vi "PID_controllerT_05.vi"() -> ()   [LabVIEW 2011]
uses:
  <vilib>/Platform/TimedLoop/XDataNode/nitl_modes.ctl
  <vilib>/Platform/TimedLoop/XDataNode/timing_clust.ctl
  <vilib>/Platform/TimedLoop/XDataNode/wakeup.ctl
  <vilib>/Platform/TimedLoop/XDataNode/XDataNode.xnode
  <vilib>/Platform/TimedLoop/XDataNode/XDNodeRunTimeDep.lvlib
panel:
  out "error(t-t0)":cluster{dbl, "Value":dbl}[](array[cluster])
  out "error":dbl
  out "tStart(s)":dbl
  out "x-y":dbl
  out "S00":dbl
  out "S10":dbl
  out "S20":dbl
  out "S11":dbl
  out "S01":dbl
  out "weight":dbl[](array[numeric])
  in  "# of points to watch":i32
  in  "tSmooth(s)":dbl=-1.0
  out "t0":dbl
  out "error(t)":cluster{dbl, "Value":dbl}[](array[cluster])
  out "error out":errorcluster
  out "first":bool=TRUE
  out "P (torr)":string
  out "XY Graph":cluster{dbl, "Value":dbl}[](graph)
  out "current value":dbl
  in  "stop":bool
  in  "Period (s)":dbl
  out "dValue":dbl
  out "derivative":dbl
  out "integral":dbl
  out "Current angle (deg)":dbl
  in  "Kd":dbl
  in  "Ki":dbl
  in  "Kp":dbl
  out "Current P (torr)":dbl
  in  "Set Point (torr)":dbl
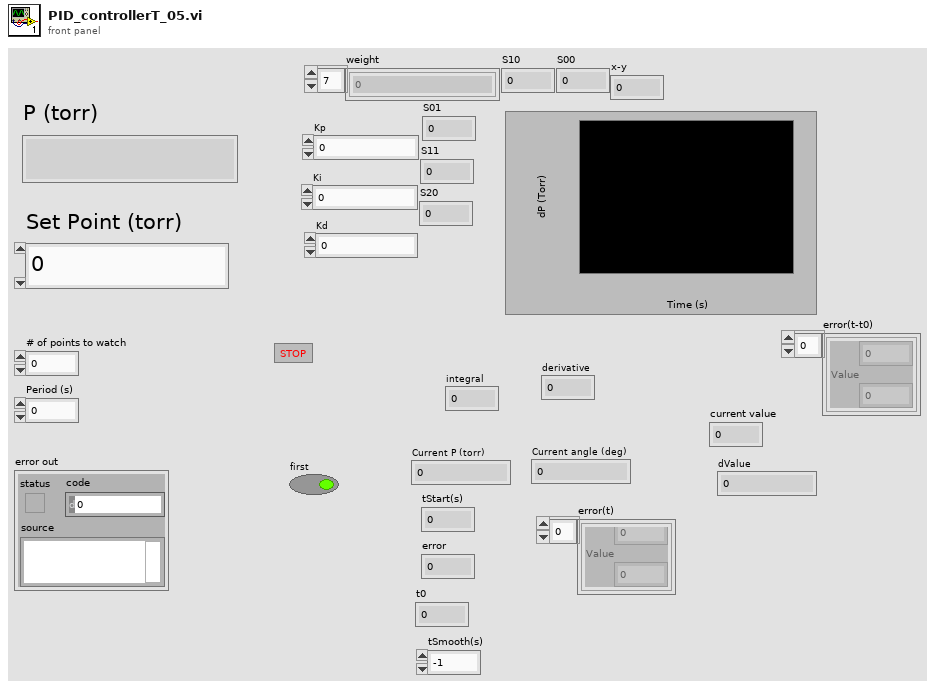
[diagram p1: front panel]
types:
  T1 = typedef "XDNodeRunTimeDep.lvlib/nitl_modes.ctl" = enum32{"No Change", "Process missed periods, maintain original phase", "Discard missed periods, maintain original phase", "Process missed periods, ignore original phase", "Discard missed periods, ignore original phase"}
  T2 = typedef "XDNodeRunTimeDep.lvlib/timing_clust.ctl" = cluster{"Expected End [f-1]":u64, "Actual End [f-1]":u64, "Finished Late? [f-1]":bool, "Expected End [i-1]":u64, "Actual End [i-1]":u64, "Finished Late? [i-1]":bool, "Expected Start [i]":u64, "Actual Start [i]":u64, "Expected Start [f]":u64, "Actual Start [f]":u64, "Source Name":string, "Structure Name":string, "Period":i64, "Deadline":i64, "Offset":i64, "Start":i64, "Priority":i32, "Timeout":i32, "Mode":T1, "Wakeup Reason":T3, "Error":errorcluster, "Source Type":string, "Secondary Source Type":string, "Global End Time":u64, "Global Start Time":u64, "Frame Duration":u64, "Iteration Duration":u64, "Assigned CPU":i32, "I/O Scan Engine Mode":u32}
  T3 = typedef "XDNodeRunTimeDep.lvlib/wakeup.ctl" = enum32{"Normal", "Aborted", "Asynchronous wakeup", "Timing source error", "Timed loop error", "Timeout"}
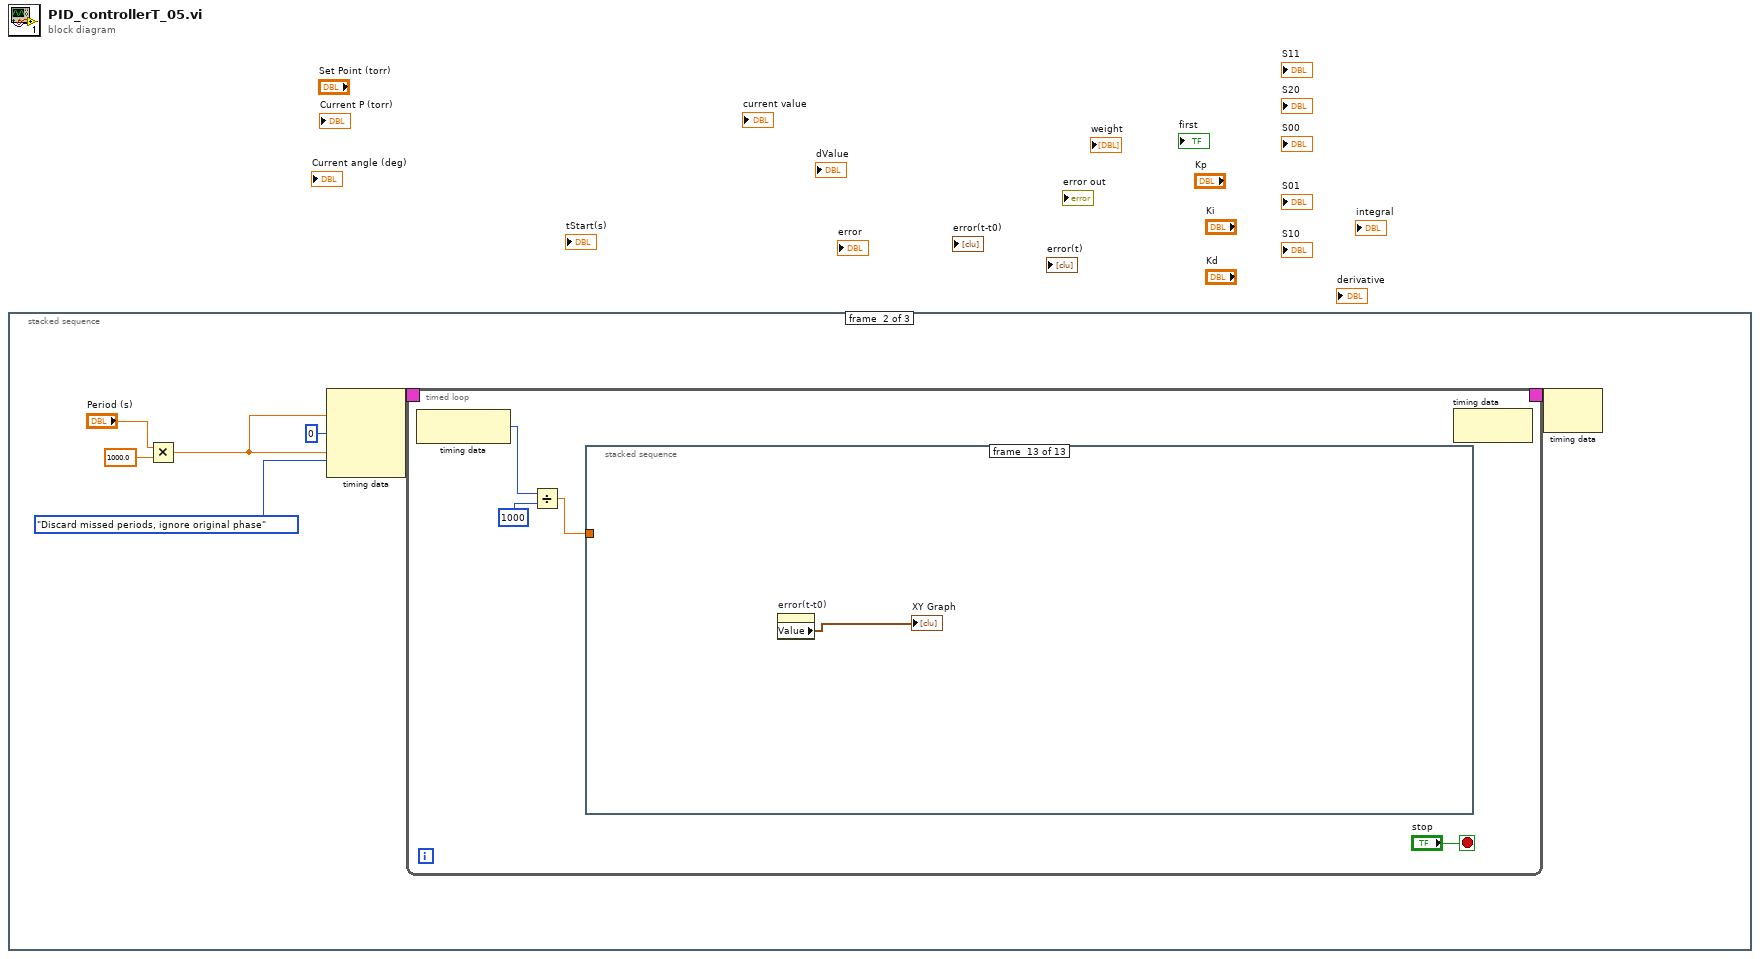
[diagram p0: block diagram]
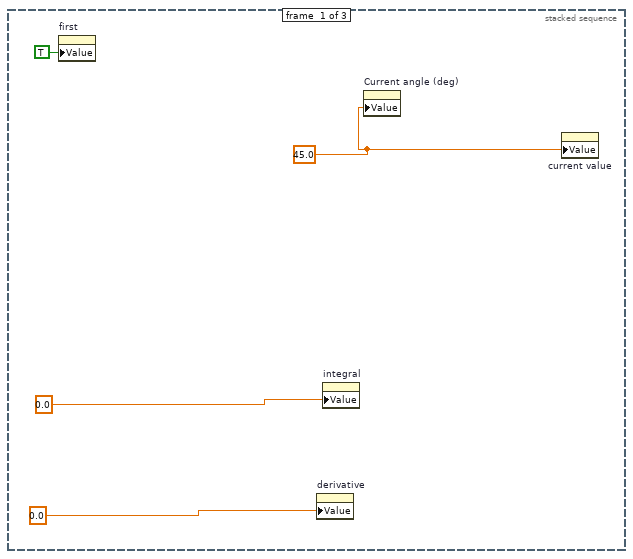
[diagram p2: hidden frame]
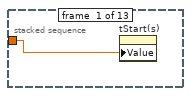
[diagram p3: hidden frame]
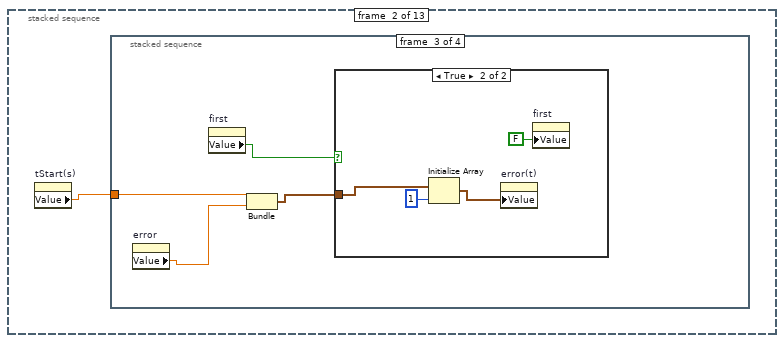
[diagram p4: hidden frame]
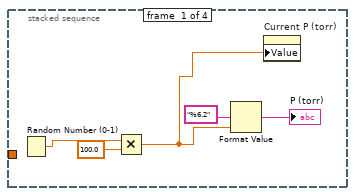
[diagram p5: hidden frame]
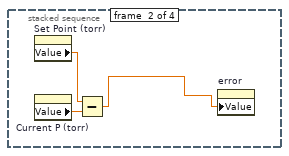
[diagram p6: hidden frame]
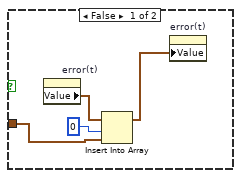
[diagram p7: hidden frame]
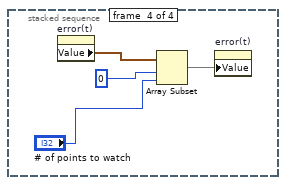
[diagram p8: hidden frame]
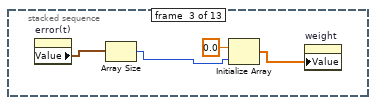
[diagram p9: hidden frame]
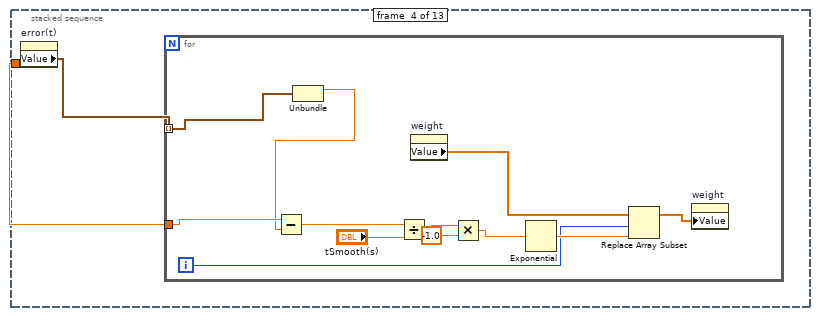
[diagram p10: hidden frame]
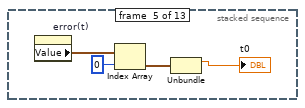
[diagram p11: hidden frame]
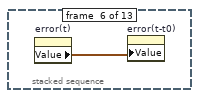
[diagram p12: hidden frame]
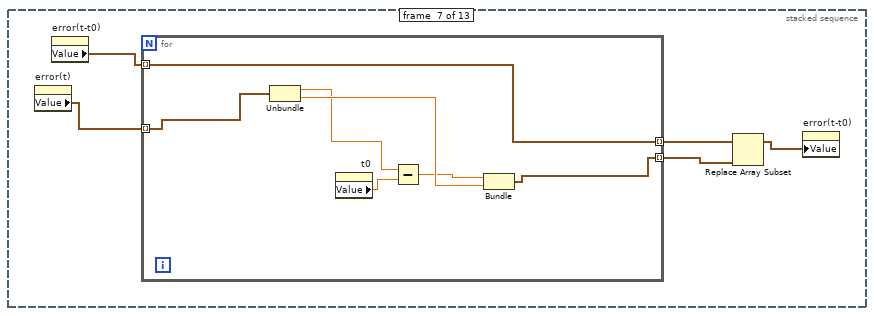
[diagram p13: hidden frame]
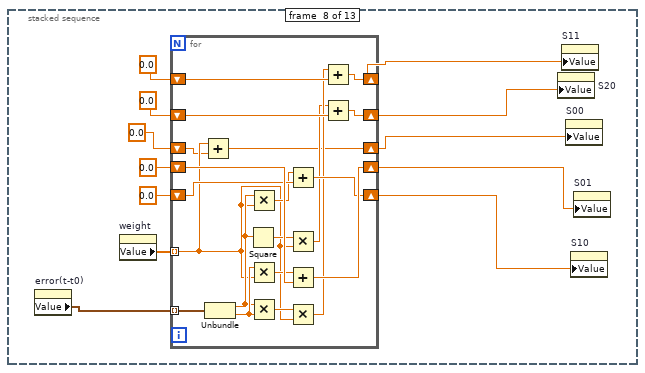
[diagram p14: hidden frame]
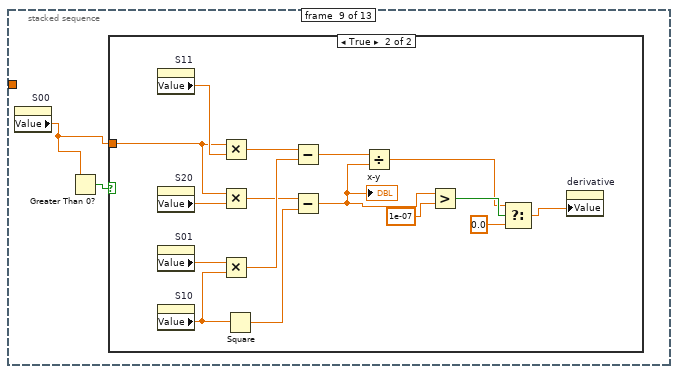
[diagram p15: hidden frame]
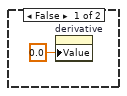
[diagram p16: hidden frame]
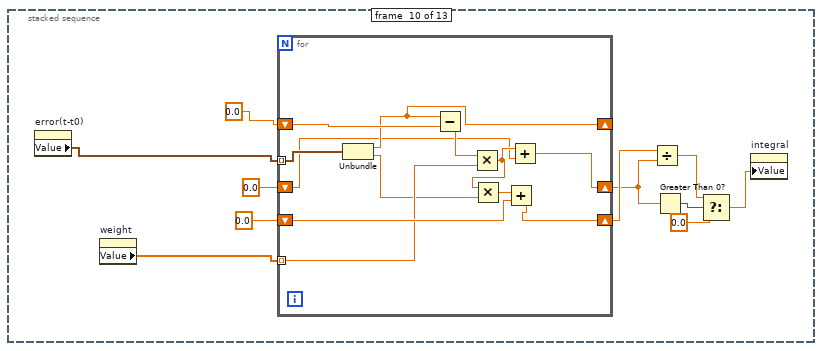
[diagram p17: hidden frame]
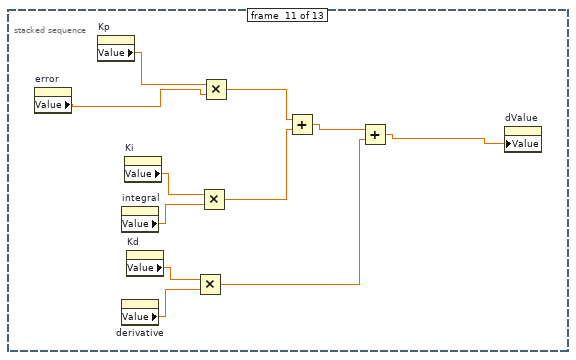
[diagram p18: hidden frame]
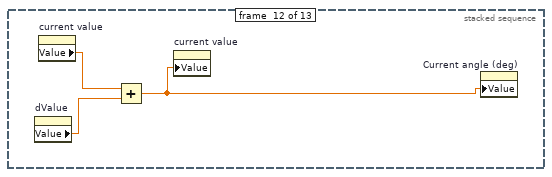
[diagram p19: hidden frame]
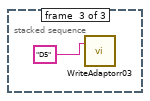
[diagram p20: hidden frame]
diagram:
  n1 = stacked-sequence {
    frame #0 {
      w1 = 45.0 ("current value")
      n2 = property on="first" class="Bool (strict)"("Value"=TRUE ("first")) -> ()  [unwired: 2 in, 2 out]
      n3 = property on="derivative" class="DigNum (strict)"("Value"=0.0 ("derivative")) -> ()  [unwired: 2 in, 2 out]
      n4 = property on="integral" class="DigNum (strict)"("Value"=0.0 ("integral")) -> ()  [unwired: 2 in, 2 out]
      n5 = property on="Current angle (deg)" class="DigNum (strict)"("Value"=w1) -> ()  [unwired: 2 in, 2 out]
      n6 = property on="current value" class="DigNum (strict)"("Value"=w1) -> ()  [unwired: 2 in, 2 out]
    }
    frame #1 {
      n7 = Multiply(x="Period (s)", y=1000.0) -> (x*y=w6:dbl)
      n8 = node-c288(w6, i64 0 ("Offset"), w6, nitl_modes."Discard missed periods, ignore original phase" ("Mode")) -> (w11:T2)
      n9 = timed-loop {
        timing: w11 -> [_]
        timing-out: [_] -> w10
        stop <- "stop" stop-if-true
        n10 = node-c288() -> (w12:i64)  [unwired: 1 in]
        n11 = Divide(x=w12, y=i64 1000) -> (x/y=w13:dbl)
        n12 = stacked-sequence {
          tunnel: w13 -> [w16 _ _ w46 _ _ _ _ _ _ _ _ _]
          frame #0 {
            n13 = property on="tStart(s)" class="DigNum (strict)"("Value"=w16) -> ()  [unwired: 2 in, 2 out]
          }
          frame #1 {
            n14 = property on="tStart(s)" class="DigNum (strict)"() -> ("Value"=w17:dbl)  [unwired: 2 in, 2 out]
            n15 = stacked-sequence {
              tunnel: w17 -> [_ _ w28 _]
              frame #0 {
                n16 = Random Number (0-1)() -> (number: 0 to 1=w19:dbl)
                n17 = Multiply(x=w19, y=100.0) -> (x*y=w18:dbl)
                n18 = Format Value(format string="%6.2", value (0)=w18) -> (output string=→"P (torr)":string)  [unwired: 1 in]
                n19 = property on="Current P (torr)" class="DigNum (strict)"("Value"=w18) -> ()  [unwired: 2 in, 2 out]
              }
              frame #1 {
                n20 = property on="Set Point (torr)" class="DigNum (strict)"() -> ("Value"=w24:dbl)  [unwired: 2 in, 2 out]
                n21 = property on="Current P (torr)" class="DigNum (strict)"() -> ("Value"=w25:dbl)  [unwired: 2 in, 2 out]
                n22 = Subtract(x=w24, y=w25) -> (x-y=w23:dbl)
                n23 = property on="error" class="DigNum (strict)"("Value"=w23) -> ()  [unwired: 2 in, 2 out]
              }
              frame #2 {
                n24 = property on="error" class="DigNum (strict)"() -> ("Value"=w26:dbl)  [unwired: 2 in, 2 out]
                n25 = property on="first" class="Bool (strict)"() -> ("Value"=w29:bool)  [unwired: 2 in, 2 out]
                n26 = Bundle("Value"=w28, "Value"=w26) -> (w27:cluster{"Value":dbl, "Value":dbl})  [unwired: 1 in]
                n27 = case shown="True" w29 {
                  tunnel: w27 -> [w31 w36]
                  frame False {
                    n28 = property on="error(t)" class="Arr (strict)"() -> ("Value"=w32:cluster{dbl, "Value":dbl}[])  [unwired: 2 in, 2 out]
                    n29 = Insert Into Array(array=w32, index=0, new element=w31) -> (w30:cluster{dbl, "Value":dbl}[])
                    n30 = property on="error(t)" class="Arr (strict)"("Value"=w30) -> ()  [unwired: 2 in, 2 out]
                  }
                  frame True {
                    n31 = Initialize Array(w36, 1 ("dimension size")) -> (w34:cluster{"Value":dbl, "Value":dbl}[])
                    n32 = property on="error(t)" class="Arr (strict)"("Value"=w34) -> ()  [unwired: 2 in, 2 out]
                    n33 = property on="first" class="Bool (strict)"("Value"=FALSE ("first")) -> ()  [unwired: 2 in, 2 out]
                  }
                }
              }
              frame #3 {
                n34 = property on="error(t)" class="Arr (strict)"() -> ("Value"=w39:cluster{dbl, "Value":dbl}[])  [unwired: 2 in, 2 out]
                n35 = Array Subset(array=w39, index=0, length="# of points to watch") -> (w41:cluster{dbl, "Value":dbl}[])
                n36 = property on="error(t)" class="Arr (strict)"("Value"=w41) -> ()  [unwired: 2 in, 2 out]
              }
            }
          }
          frame #2 {
            n37 = property on="error(t)" class="Arr (strict)"() -> ("Value"=w45:cluster{dbl, "Value":dbl}[])  [unwired: 2 in, 2 out]
            n38 = Array Size(array=w45) -> (size(s)=w43:i32)
            n39 = Initialize Array(0.0 ("element"), w43) -> (w42:dbl[])
            n40 = property on="weight" class="Arr (strict)"("Value"=w42) -> ()  [unwired: 2 in, 2 out]
          }
          frame #3 {
            n41 = property on="error(t)" class="Arr (strict)"() -> ("Value"=w47:cluster{dbl, "Value":dbl}[])  [unwired: 2 in, 2 out]
            n42 = for {
              tunnel: w47 -> [w59] mode=indexing
              tunnel: w46 -> [w58]
              i -> [w54]
              n43 = Unbundle(w59) -> (w57:dbl)  [unwired: 1 out]
              n44 = Subtract(x=w58, y=w57) -> (x-y=w52:dbl)
              n45 = Divide(x=w52, y="tSmooth(s)") -> (x/y=w50:dbl)
              n46 = property on="weight" class="Arr (strict)"() -> ("Value"=w55:dbl[])  [unwired: 2 in, 2 out]
              n47 = Multiply(x=w50, y=-1.0) -> (x*y=w48:dbl)
              n48 = Exponential(1:w48) -> (0:w56:dbl)
              n49 = Replace Array Subset(array=w55, new element=w56, index=w54) -> (w53:dbl[])
              n50 = property on="weight" class="Arr (strict)"("Value"=w53) -> ()  [unwired: 2 in, 2 out]
            }
          }
          frame #4 {
            n51 = property on="error(t)" class="Arr (strict)"() -> ("Value"=w63:cluster{dbl, "Value":dbl}[])  [unwired: 2 in, 2 out]
            n52 = Index Array(array=w63, index=0) -> (element=w61:cluster{dbl, "Value":dbl})
            n53 = Unbundle(w61) -> (→"t0":dbl)  [unwired: 1 out]
          }
          frame #5 {
            n54 = property on="error(t)" class="Arr (strict)"() -> ("Value"=w64:cluster{dbl, "Value":dbl}[])  [unwired: 2 in, 2 out]
            n55 = property on="error(t-t0)" class="Arr (strict)"("Value"=w64) -> ()  [unwired: 2 in, 2 out]
          }
          frame #6 {
            n56 = property on="error(t)" class="Arr (strict)"() -> ("Value"=w69:cluster{dbl, "Value":dbl}[])  [unwired: 2 in, 2 out]
            n57 = property on="error(t-t0)" class="Arr (strict)"() -> ("Value"=w67:cluster{dbl, "Value":dbl}[])  [unwired: 2 in, 2 out]
            n58 = for {
              tunnel: w69 -> [w72] mode=indexing
              tunnel: [w71] -> w68 mode=indexing
              tunnel: w67 -> [w70] mode=indexing
              tunnel: [w70] -> w66 mode=indexing
              n59 = Unbundle(w72) -> (w73:dbl, "Value"=w75:dbl)
              n60 = property on="t0" class="DigNum (strict)"() -> ("Value"=w76:dbl)  [unwired: 2 in, 2 out]
              n61 = Subtract(x=w73, y=w76) -> (x-y=w74:dbl)
              n62 = Bundle(w74, "Value"=w75) -> (w71:cluster{dbl, "Value":dbl})  [unwired: 1 in]
            }
            n63 = Replace Array Subset(array=w66, new element=w68) -> (w65:cluster{dbl, "Value":dbl}[])  [unwired: 1 in]
            n64 = property on="error(t-t0)" class="Arr (strict)"("Value"=w65) -> ()  [unwired: 2 in, 2 out]
          }
          frame #7 {
            n65 = property on="error(t-t0)" class="Arr (strict)"() -> ("Value"=w77:cluster{dbl, "Value":dbl}[])  [unwired: 2 in, 2 out]
            n66 = property on="weight" class="Arr (strict)"() -> ("Value"=w84:dbl[])  [unwired: 2 in, 2 out]
            n67 = for {
              tunnel: w77 -> [w104] mode=indexing
              shift-right: [w105] -> w79
              shift-left: 0.0 -> [w108]
              shift-right: [w101] -> w82
              shift-left: 0.0 -> [w107]
              shift-right: [w100] -> w81
              shift-left: 0.0 -> [w106]
              shift-right: [w102] -> w78
              shift-left: 0.0 -> [w103]
              tunnel: w84 -> [w91] mode=indexing
              shift-right: [w89] -> w80
              shift-left: 0.0 -> [w90]
              n68 = Add(x=w91, y=w90) -> (x+y=w89:dbl)
              n69 = Unbundle(w104) -> (w93:dbl, "Value"=w99:dbl)
              n70 = Square(x=w93) -> (x^2=w95:dbl)
              n71 = Multiply(x=w93, y=w91) -> (x*y=w92:dbl)
              n72 = Multiply(x=w99, y=w91) -> (x*y=w98:dbl)
              n73 = Multiply(x=w93, y=w99) -> (x*y=w97:dbl)
              n74 = Add(x=w92, y=w103) -> (x+y=w102:dbl)
              n75 = Multiply(x=w95, y=w91) -> (x*y=w94:dbl)
              n76 = Add(x=w98, y=w108) -> (x+y=w105:dbl)
              n77 = Multiply(x=w97, y=w91) -> (x*y=w96:dbl)
              n78 = Add(x=w96, y=w107) -> (x+y=w101:dbl)
              n79 = Add(x=w94, y=w106) -> (x+y=w100:dbl)
            }
            n80 = property on="S20" class="DigNum (strict)"("Value"=w81) -> ()  [unwired: 2 in, 2 out]
            n81 = property on="S11" class="DigNum (strict)"("Value"=w82) -> ()  [unwired: 2 in, 2 out]
            n82 = property on="S00" class="DigNum (strict)"("Value"=w80) -> ()  [unwired: 2 in, 2 out]
            n83 = property on="S10" class="DigNum (strict)"("Value"=w78) -> ()  [unwired: 2 in, 2 out]
            n84 = property on="S01" class="DigNum (strict)"("Value"=w79) -> ()  [unwired: 2 in, 2 out]
          }
          frame #8 {
            n85 = property on="S00" class="DigNum (strict)"() -> ("Value"=w109:dbl)  [unwired: 2 in, 2 out]
            n86 = Greater Than 0?(x=w109) -> (x > 0?=w110:bool)
            n87 = case shown="True" w110 {
              tunnel: w109 -> [_ w119]
              frame False {
                n88 = property on="derivative" class="DigNum (strict)"("Value"=0.0 ("derivative")) -> ()  [unwired: 2 in, 2 out]
              }
              frame True {
                n89 = property on="S11" class="DigNum (strict)"() -> ("Value"=w121:dbl)  [unwired: 2 in, 2 out]
                n90 = property on="S20" class="DigNum (strict)"() -> ("Value"=w120:dbl)  [unwired: 2 in, 2 out]
                n91 = property on="S01" class="DigNum (strict)"() -> ("Value"=w118:dbl)  [unwired: 2 in, 2 out]
                n92 = property on="S10" class="DigNum (strict)"() -> ("Value"=w122:dbl)  [unwired: 2 in, 2 out]
                n93 = Multiply(x=w119, y=w121) -> (x*y=w127:dbl)
                n94 = Multiply(x=w119, y=w120) -> (x*y=w125:dbl)
                n95 = Multiply(x=w118, y=w122) -> (x*y=w126:dbl)
                n96 = Square(x=w122) -> (x^2=w124:dbl)
                n97 = Subtract(x=w127, y=w126) -> (x-y=w123:dbl)
                n98 = Subtract(x=w125, y=w124) -> (x-y=w117:dbl)
                "x-y" <- w117
                n99 = Divide(x=w123, y=w117) -> (x/y=w113:dbl)
                n100 = Greater?(x=w117, y=1e-07) -> (0:w115:bool)
                n101 = Select(t=w113, s=w115, f=0.0) -> (s? t:f=w114:dbl)
                n102 = property on="derivative" class="DigNum (strict)"("Value"=w114) -> ()  [unwired: 2 in, 2 out]
              }
            }
          }
          frame #9 {
            n103 = property on="error(t-t0)" class="Arr (strict)"() -> ("Value"=w128:cluster{dbl, "Value":dbl}[])  [unwired: 2 in, 2 out]
            n104 = property on="weight" class="Arr (strict)"() -> ("Value"=w137:dbl[])  [unwired: 2 in, 2 out]
            n105 = for {
              tunnel: w128 -> [w150] mode=indexing
              shift-right: [w148] -> _
              shift-left: 0.0 -> [w149]
              tunnel: w137 -> [w143] mode=indexing
              shift-right: [w144] -> w134
              shift-left: 0.0 -> [w145]
              shift-right: [w140] -> w133
              shift-left: 0.0 -> [w139]
              n106 = Unbundle(w150) -> (w148:dbl, "Value"=w142:dbl)
              n107 = Subtract(x=w148, y=w149) -> (x-y=w147:dbl)
              n108 = Multiply(x=w147, y=w143) -> (x*y=w141:dbl)
              n109 = Multiply(x=w141, y=w142) -> (x*y=w146:dbl)
              n110 = Add(x=w146, y=w145) -> (x+y=w144:dbl)
              n111 = Add(x=w141, y=w139) -> (x+y=w140:dbl)
            }
            n112 = Divide(x=w134, y=w133) -> (x/y=w131:dbl)
            n113 = Greater Than 0?(x=w133) -> (x > 0?=w132:bool)
            n114 = Select(t=w131, s=w132, f=0.0) -> (s? t:f=w129:dbl)
            n115 = property on="integral" class="DigNum (strict)"("Value"=w129) -> ()  [unwired: 2 in, 2 out]
          }
          frame #10 {
            n116 = property on="error" class="DigNum (strict)"() -> ("Value"=w151:dbl)  [unwired: 2 in, 2 out]
            n117 = property on="Kp" class="DigNum (strict)"() -> ("Value"=w161:dbl)  [unwired: 2 in, 2 out]
            n118 = property on="integral" class="DigNum (strict)"() -> ("Value"=w159:dbl)  [unwired: 2 in, 2 out]
            n119 = property on="derivative" class="DigNum (strict)"() -> ("Value"=w157:dbl)  [unwired: 2 in, 2 out]
            n120 = property on="Ki" class="DigNum (strict)"() -> ("Value"=w160:dbl)  [unwired: 2 in, 2 out]
            n121 = property on="Kd" class="DigNum (strict)"() -> ("Value"=w158:dbl)  [unwired: 2 in, 2 out]
            n122 = Multiply(x=w158, y=w157) -> (x*y=w154:dbl)
            n123 = Multiply(x=w160, y=w159) -> (x*y=w155:dbl)
            n124 = Multiply(x=w161, y=w151) -> (x*y=w156:dbl)
            n125 = Add(x=w156, y=w155) -> (x+y=w153:dbl)
            n126 = Add(x=w153, y=w154) -> (x+y=w152:dbl)
            n127 = property on="dValue" class="DigNum (strict)"("Value"=w152) -> ()  [unwired: 2 in, 2 out]
          }
          frame #11 {
            n128 = property on="dValue" class="DigNum (strict)"() -> ("Value"=w163:dbl)  [unwired: 2 in, 2 out]
            n129 = property on="current value" class="DigNum (strict)"() -> ("Value"=w164:dbl)  [unwired: 2 in, 2 out]
            n130 = Add(x=w164, y=w163) -> (x+y=w162:dbl)
            n131 = property on="current value" class="DigNum (strict)"("Value"=w162) -> ()  [unwired: 2 in, 2 out]
            n132 = property on="Current angle (deg)" class="DigNum (strict)"("Value"=w162) -> ()  [unwired: 2 in, 2 out]
          }
          frame #12 {
            n133 = property on="error(t-t0)" class="Arr (strict)"() -> ("Value"=→"XY Graph":cluster{dbl, "Value":dbl}[])  [unwired: 2 in, 2 out]
          }
        }
        n134 = node-c288() -> ()  [unwired: 1 in, 1 out]
      }
      n135 = node-c288(w10) -> ()  [unwired: 1 out]
    }
    frame #2 {
      n136 = call "WriteAdaptorr03.vi"("string to write"="D5") -> ()  [unwired: 1 in, 1 out]
    }
  }
